vi "Voltage input PID Autotuning Offline.vi"() -> ()   [LabVIEW 2019]
uses:
  <vilib>/addons/control/pid/pid.llb/PID Advanced (DBL).vi
  <vilib>/addons/control/pid/autopid.llb/PID Autotuning Design (Ziegler-Nichols).vi
  <vilib>/addons/control/pid/autopid.llb/PID Autotuning Design (Cohen-Coon).vi
  <vilib>/addons/control/pid/autopid.llb/PID Autotuning Design (Chien-Hrones-Reswick).vi
  <vilib>/addons/control/pid/autopid.llb/PID Autotuning Design (Internal Model Control).vi
  <vilib>/addons/control/pid/NI_PID_pid.lvlib
  <vilib>/ptbypt/NI_PtbyPt.lvlib
  <vilib>/addons/control/pid/NI_PID_autopid.lvlib
  <vilib>/measure/NI_MABase.lvlib
panel:
  out "MSE":dbl(graph)
  out "mse":dbl format="%0.2f"
  in  "reset signal":bool
  in  "offset":dbl=5.0 format="%0.2p"
  in  "sampling info":cluster{"Fs":dbl, "#s":dbl}={"Fs"=1000.0, "#s"=1000.0}
  in  "phase":dbl format="%.2p"
  in  "amplitude":dbl=5.0 format="%0.2p"
  in  "frequency":dbl=0.01 format="%#.6g"
  in  "signal type":T1(ring)
  out "Valve input voltage":dbl(graph)
  in  "Tab Control":T2(tab)
  in  "Instructions":string="Overview: This example demonstrates how to use the PID Autotuning Design to obtain PID parameters based on setpoint and process variable collected in another loop.\nInstructions:\n1. Run the VI and wait until the process variable (PV) reaches near setpoint (SP).\n2.  In the PID Autotuning Design section, select the type of algorithm, type of controller and excitation amplitude for the 'open loop step response'. Then, click Autotune to start the process. Select the Identified Plant Parameter tab and see the results from the identification.\n3.  When the tuned PID gains do not change anymore, the identification is done and you have the option to accept by clicking Accept gain, which will transfer the new gain to PID Gains.\n4. Click the Autotune button again to go back to the automatic control state. You can try different options and repeat this process.\n5. Click Stop to stop the VI.\n"
  out "Identified Plant Parameters":T3={"Plant Gain (K)"=1.7609511324977591, "Time Constant (T)"=1.9621978490901302, "Dead Time (L)"=0.22467425343567116}
  out "Control Output":dbl[](graph)
  out "Measurement":dbl[](graph)
  out "Stimulus operating point":dbl=20.314221540357543
  out "Response operating point":dbl=51.08345461694337
  out "Tuned PID gains":T4={"proportional gain (Kc)"=1.9838195929127882, "integral time (Ti, min)"=0.01995856284686879, "derivative time (Td, min)"=0.0} {"derivative time (Td, min)" format="%#.6g"; "integral time (Ti, min)" format="%#.6g"; "proportional gain (Kc)" format="%#.6g"}
  in  "Accept gain":bool
  in  "Control":T5(tab)
  in  "Ziegler-Nichols speed":u16(ring) items=["Fast", "Normal", "Slow"]
  in  "Tuning specifications":u16(ring) items=["Regulator - 0 %", "Regulator -  20%", "Servo - 0%", "Servo - 20%"]
  in  "Multiplicative factor":dbl(slide)=1.0 scale=0.01..100.0
  in  "Type of controller":u16(ring)=2 items=["P", "PI", "PID"]
  in  "Stop":bool
  out "SP and PV":cluster{"initial PV":dbl, "SP1:":dbl}(graph)={"initial PV"=50.98160323470328, "SP1:"=50.98039215686275}
  in  "Sampling Time dt (s)":dbl=0.05 min=0.001 step=0.01 format="%#.3p"
  in  "PID Gains":T4={"proportional gain (Kc)"=5.0, "integral time (Ti, min)"=0.2, "derivative time (Td, min)"=0.0} {"derivative time (Td, min)" format="%#.6g"; "integral time (Ti, min)" format="%#.6g"; "proportional gain (Kc)" format="%#.6g"}
  out "PV:":dbl(slide)=50.98160323470328 scale=0.0..10.0
  in  "Autotune":bool
  out "MV":dbl(graph)=20.39115328927357
  in  "Reinitialize":bool
  in  "Excitation":dbl=0.5 format="%.2f"
  in  "Automatic":bool=TRUE
  in  "MV:":dbl(slide)=20.39115328927357 scale=-100.0..100.0
  # "No additional parameters"
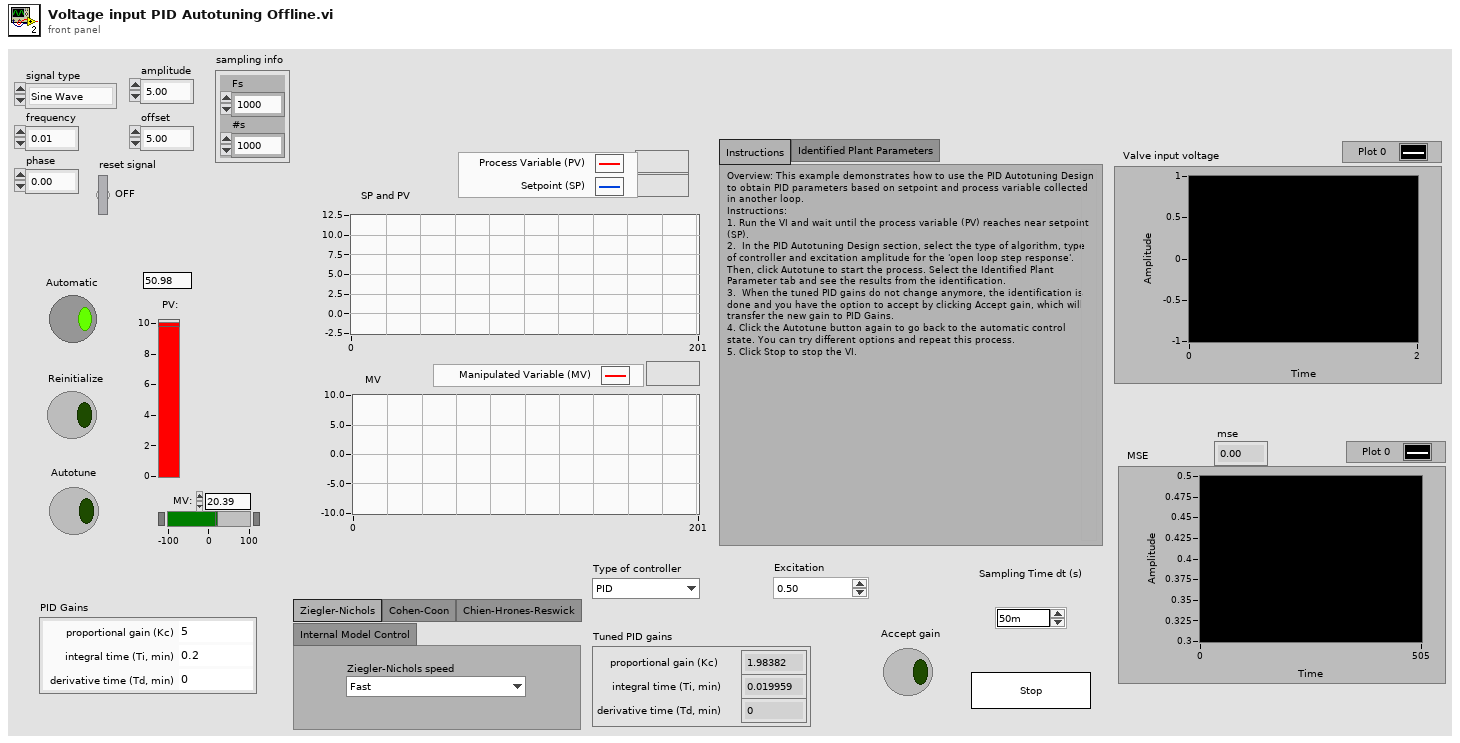
[diagram p1: front panel]
types:
  T1 = enum16{"Sine Wave", "Triangle Wave", "Square Wave", "Sawtooth Wave"}
  T2 = enum32{"Instructions", "Identified Plant Parameters"}
  T3 = cluster{"Plant Gain (K)":dbl, "Time Constant (T)":dbl, "Dead Time (L)":dbl}
  T4 = cluster{"proportional gain (Kc)":dbl, "integral time (Ti, min)":dbl, "derivative time (Td, min)":dbl}
  T5 = enum32{"Ziegler-Nichols", "Cohen-Coon", "Chien-Hrones-Reswick", "Internal Model Control"}
  T6 = cluster{"static gain":dbl, "lag (s)":dbl, "deadtime (s)":dbl, "load":dbl, "deadband":dbl, "sensor noise":dbl, "initial PV":dbl, "plant noise":dbl}
  T7 = cluster{"Voltage":dbl, "signal out":waveform(dbl)}
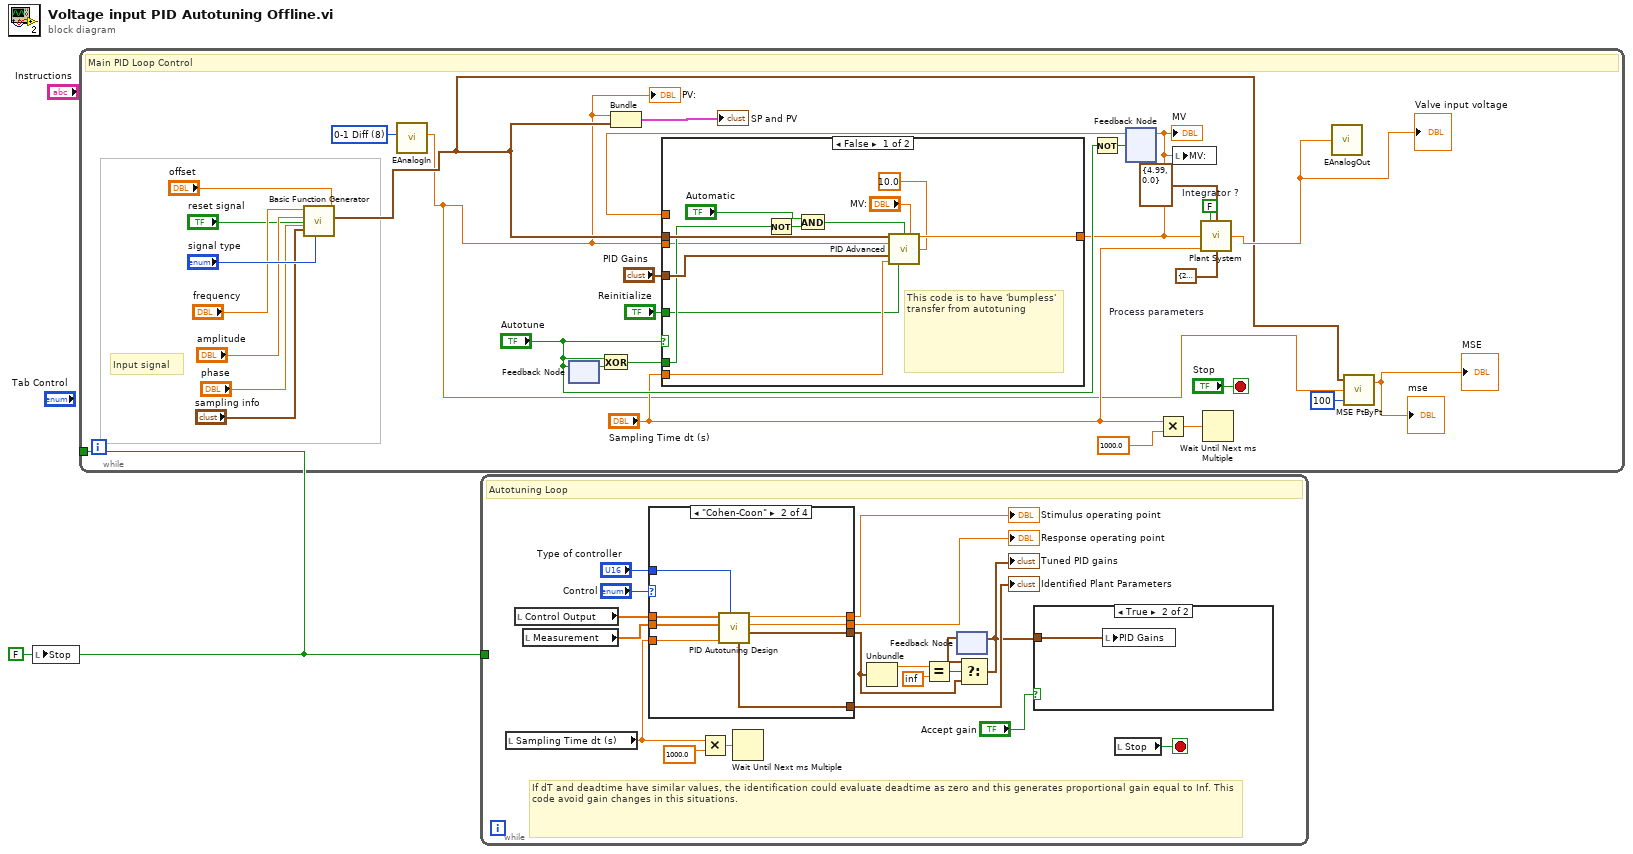
[diagram p0: block diagram]
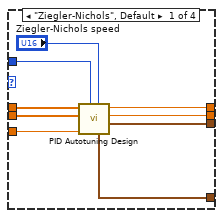
[diagram p2: hidden frame]
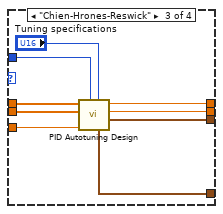
[diagram p3: hidden frame]
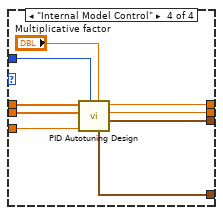
[diagram p4: hidden frame]
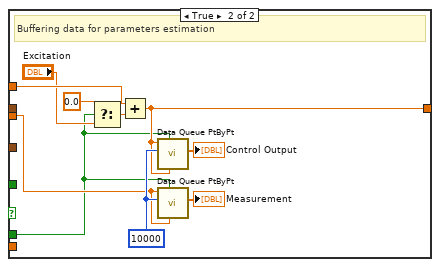
[diagram p6: hidden frame]
diagram:
  w1 = FALSE ("Stop")
  n1 = local write "Stop"(w1) -> ()
  n2 = while {
    tunnel: w1 -> [_]
    stop <- "Stop" stop-if-true
    w13 = u16 8 items=["0 SE (+/-10V)", "1 SE (+/-10V)", "2 SE (+/-10V)", "3 SE (+/-10V)", "4 SE (+/-10V)", "5 SE (+/-10V)", "6 SE (+/-10V)", "7 SE (+/-10V)", "0-1 Diff", "2-3 Diff", "4-5 Diff", "6-7 Diff"] ("Channel")
    w20 = T6 {"static gain"=2.5, "lag (s)"=2.5, "deadtime (s)"=0.01, "load"=0.0, "deadband"=0.0, "sensor noise"=0.0, "initial PV"=30.0, "plant noise"=0.0}  # Process parameters
    w21 = FALSE  # Integrator ?
    # "Input signal"
    # "Main PID Loop Control"
    n3 = call <vilib>:"Basic Function Generator.vi"("offset"="offset", "reset signal"="reset signal", "sampling info"="sampling info", "signal type"="signal type", "phase"="phase", "amplitude"="amplitude", "frequency"="frequency") -> ("signal out"=w5:waveform(dbl))  [unwired: 2 in, 2 out]
    n4 = call <vilib>:"EAnalogIn.vi"("Channel"=w13) -> ("Voltage"=w4:dbl)  [unwired: 6 in, 4 out]
    "PV:" <- w4
    n5 = feedback #1() -> (w26:bool)  [unwired: 1 in]
    n6 = feedback-in #1("Autotune") -> ()
    n7 = Exclusive Or(1:w26, 2:"Autotune") -> (0:w25:bool)
    n8 = Bundle("Voltage"=w4, "signal out"=w5) -> (→"SP and PV":T7)  [unwired: 1 in]
    n9 = Not(x="Autotune") -> (.not. x?=w22:bool)
    n10 = feedback #2() -> (w24:dbl)  [unwired: 1 in]
    n11 = case shown="False" "Autotune" {
      tunnel: "Sampling Time dt (s)" -> [w42 _]
      tunnel: [w40 w45] -> w19
      tunnel: w4 -> [w37 w44]
      tunnel: w5 -> [w39 _]
      tunnel: "PID Gains" -> [w41 _]
      tunnel: "Reinitialize" -> [w35 _]
      tunnel: w25 -> [w38 w43]
      tunnel: w24 -> [_ w49]
      frame False {
        # "This code is to have 'bumpless' transfer from autotuning"
        n12 = Not(x=w38) -> (.not. x?=w34:bool)
        n13 = And(x="Automatic", y=w34) -> (x .and. y?=w36:bool)
        n14 = call-poly <vilib>:"PID Advanced.vi"("setpoint"=w39, "auto? (T)"=w36, "manual control"="MV:", "process variable"=w37, "alpha"=10.0, "PID gains"=w41, "dt (s)"=w42, "reinitialize? (F)"=w35) -> ("output"=w40:dbl)  [unwired: 6 in, 1 out]
      }
      frame True {
        w52 = 10000 ("sample length")
        # "Buffering data for parameters estimation"
        n15 = Select(t=0.0, s=w43, f="Excitation") -> (s? t:f=w50:dbl)
        n16 = Add(x=w49, y=w50) -> (x+y=w45:dbl)
        n17 = call <vilib>:"Data Queue PtByPt.vi"("initial queue element"=w45, "initialize"=w43, "sample length"=w52, "input data point"=w45) -> ("Current Queue"=→"Control Output":dbl[])  [unwired: 3 in, 4 out]
        n18 = call <vilib>:"Data Queue PtByPt.vi"("initial queue element"=w44, "initialize"=w43, "sample length"=w52, "input data point"=w44) -> ("Current Queue"=→"Measurement":dbl[])  [unwired: 3 in, 4 out]
      }
    }
    "MV" <- w19
    n19 = feedback-in #2(w19, w22) -> ()
    n20 = Multiply(x="Sampling Time dt (s)", y=1000.0) -> (x*y=w17:dbl)
    n21 = local write "MV:"(w19) -> ()
    n22 = call "Plant System.vi"("Integrator ?"=w21, "output saturation range"=cluster{"output high":dbl, "output low":dbl} {"output high"=4.99, "output low"=0.0}, "Plant Input"=w19, "dt (s)"="Sampling Time dt (s)", "process parameters"=w20) -> ("Plant Output"=w14:dbl)  [unwired: 10 in]
    "Valve input voltage" <- w14
    n23 = Wait Until Next ms Multiple(millisecond multiple=w17) -> ()  [unwired: 1 out]
    n24 = call <vilib>:"EAnalogOut.vi"("Analog Output 0 [volts]"=w14) -> ()  [unwired: 13 in, 2 out]
    n25 = call <vilib>:"MSE PtByPt.vi"("sample length"=100, "y"=w4, "x"=w5) -> ("mse"=→"mse" →"MSE":dbl)  [unwired: 1 in, 1 out]
  }
  n26 = while {
    tunnel: w1 -> [_]
    stop <- w65 stop-if-true
    # "If dT and deadtime have similar values, the identification could evaluate deadtime as zero and this generates proportional gain equal to Inf. This code avoid gain changes in this situations."
    # "Autotuning Loop"
    n27 = local read "Sampling Time dt (s)"() -> (w66:dbl)
    n28 = local read "Control Output"() -> (w70:dbl[])
    n29 = local read "Measurement"() -> (w69:dbl[])
    n30 = case shown="\"Cohen-Coon\"" "Control" {
      tunnel: w70 -> [w79 w87 w96 w105]
      tunnel: w69 -> [w78 w86 w95 w104]
      tunnel: [w77 w85 w94 w103] -> w68
      tunnel: [w76 w84 w93 w102] -> w67
      tunnel: w66 -> [w75 w83 w92 w101]
      tunnel: [w74 w82 w91 w100] -> w63
      tunnel: [w73 w81 w90 w99] -> w54
      tunnel: "Type of controller" -> [w72 w80 w89 w98]
      frame "Ziegler-Nichols", Default {
        n31 = call-poly <vilib>:"PID Autotuning Design.vi"("Ziegler-Nichols Speed"="Ziegler-Nichols speed", "Type of Controller"=w72, "dt (s)"=w75, "Response signal"=w78, "Stimulus signal"=w79) -> ("PID gains"=w73:T4, "response operating point"=w76:dbl, "stimulus operating point"=w77:dbl, "Plant Parameters"=w74:T3)  [unwired: 3 in]
      }
      frame "Cohen-Coon" {
        n32 = call-poly <vilib>:"PID Autotuning Design.vi"("Type of Controller"=w80, "dt (s)"=w83, "Response signal"=w86, "Stimulus signal"=w87) -> ("PID gains"=w81:T4, "response offset"=w84:dbl, "stimulus offset"=w85:dbl, "Plant Parameters"=w82:T3)  [unwired: 4 in]
      }
      frame "Chien-Hrones-Reswick" {
        n33 = call-poly <vilib>:"PID Autotuning Design.vi"("Tuning specifications"="Tuning specifications", "Type of Controller"=w89, "dt (s)"=w92, "Response signal"=w95, "Stimulus signal"=w96) -> ("PID gains"=w90:T4, "response offset"=w93:dbl, "stimulus offset"=w94:dbl, "Plant Parameters"=w91:T3)  [unwired: 3 in]
      }
      frame "Internal Model Control" {
        n34 = call-poly <vilib>:"PID Autotuning Design.vi"("Desired Time Constant (tau_c)"="Multiplicative factor", "Type of Controller"=w98, "dt (s)"=w101, "Response signal"=w104, "Stimulus signal"=w105) -> ("PID gains"=w99:T4, "response offset"=w102:dbl, "stimulus offset"=w103:dbl, "Plant Parameters"=w100:T3)  [unwired: 3 in]
      }
    }
    "Stimulus operating point" <- w68
    "Response operating point" <- w67
    "Identified Plant Parameters" <- w63
    n35 = Multiply(x=w66, y=1000.0) -> (x*y=w62:dbl)
    n36 = Wait Until Next ms Multiple(millisecond multiple=w62) -> ()  [unwired: 1 out]
    n37 = Unbundle(w54) -> ("proportional gain (Kc)"=w57:dbl)  [unwired: 2 out]
    n38 = Equal?(x=w57, y=inf) -> (x = y?=w56:bool)
    n39 = feedback #3() -> (w55:T4)  [unwired: 1 in]
    n40 = Select(t=w55, s=w56, f=w54) -> (s? t:f=w53:T4)
    "Tuned PID gains" <- w53
    n41 = feedback-in #3(w53) -> ()
    n42 = case shown="True" "Accept gain" {
      tunnel: w53 -> [_ w106]
      frame False {
      }
      frame True {
        n43 = local write "PID Gains"(w106) -> ()
      }
    }
    n44 = local read "Stop"() -> (w65:bool)
  }
